vi "Untitled 4.vi"() -> ()   [LabVIEW 2020, in "PLCMonitor.lvlib"]
uses:
  PLCMonitor/PLCMonitor.lvlib
panel:
  in  "length":u16
  in  "Start address":string
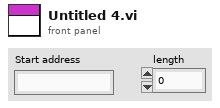
[diagram p1: front panel]
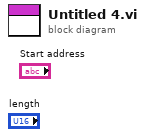
[diagram p0: block diagram]
diagram:
